vi "displayApplicationControls.vi"(10 "viewThisComponent":refnum<class "ViewThisComponent.lvclass">) -> ()   [LabVIEW 2016, in "EXAViewElements.lvlib"]
doc: "Displays application controls."
uses:
  EXAViewElements.lvlib
  ViewThisComponent/ViewThisComponent.lvclass
  home/andres/ct_cmpuserevents/ComponentTemplateCore/ComponentModel/ComponentModel/View/View.lvclass
  ComponentTemplateCore/ComponentModel/ComponentModel/Typedefs/ComponentStateValues.ctl
  Typedefs/SubDataSV.ctl
  Typedefs/EXATypedefs.lvlib
  ComponentTemplateCore/ComponentModel/ComponentModel/View/View.lvclass
panel:
  in  "Label":string(combo)
  in  "StartIsTrue":bool caption="Start"
  in  "ExitIsTrue":bool caption="Exit"
  in  "enableIsTrue":bool caption="Enable Motion"
  in  "ClearErrorIsTrue":bool caption="Clear Error"
  in  "disableIsTrue":bool caption="Disable Motion"
  in  "GoToStandbyIsTrue":bool caption="Go To Standby"
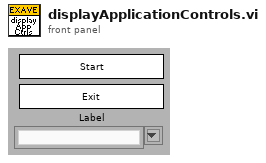
[diagram p1: front panel]
types:
  T1 = typedef "EXATypedefs.lvlib/PubDataEvents.ctl" = cluster{"DetailedState":refnum<user-event>, "ErrorCode":refnum<user-event>, "Heartbeat":refnum<user-event>, "LoopTime_ms":refnum<user-event>, "LoopTimeOutOfRange":refnum<user-event>, "RejectedCommand":refnum<user-event>, "SummaryState":refnum<user-event>, "Timestamp":refnum<user-event>, "AppliedSettingsMatchStart":refnum<user-event>, "SettingsApplied":refnum<user-event>, "SettingVersions":refnum<user-event>}
  T2 = typedef "ComponentStateValues.ctl" = enum16{"Off", "Standby", "Disabled", "Enabled", "Fault"}
  T3 = typedef "EXATypedefs.lvlib/SubDataSV.ctl" = enum16{"ClearError", "Disable", "Enable", "Exit", "GoToStandby", "HeartbeatIn", "Start"}
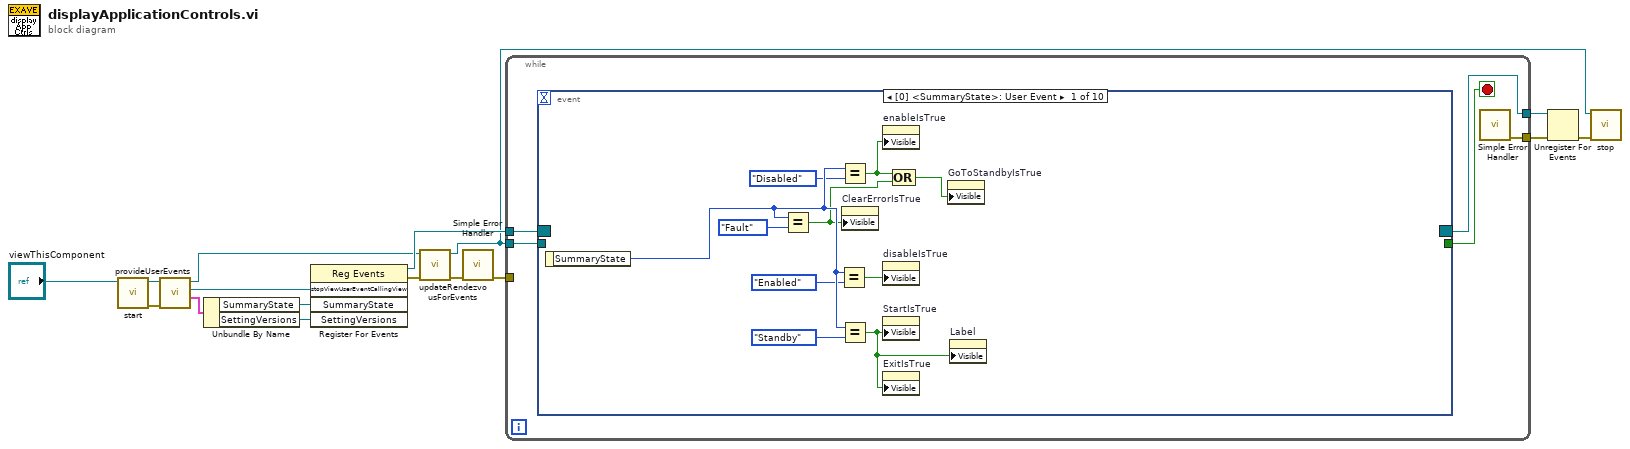
[diagram p0: block diagram]
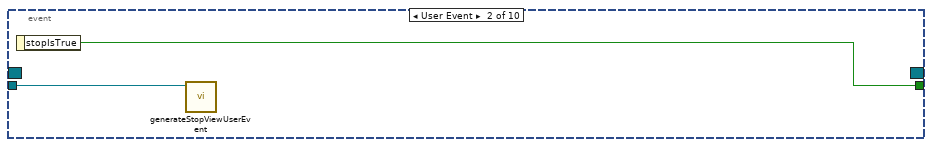
[diagram p2: hidden frame]
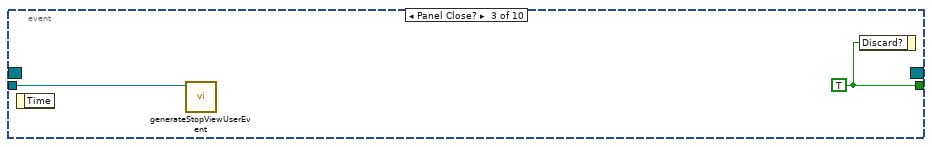
[diagram p3: hidden frame]
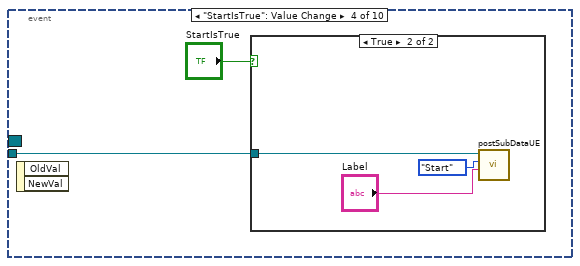
[diagram p4: hidden frame]
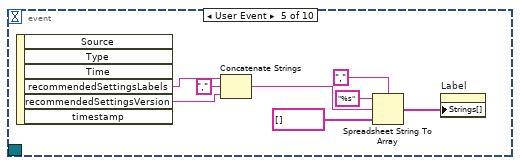
[diagram p6: hidden frame]
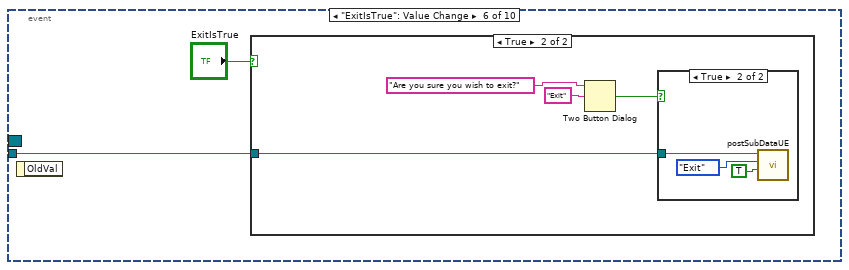
[diagram p7: hidden frame]
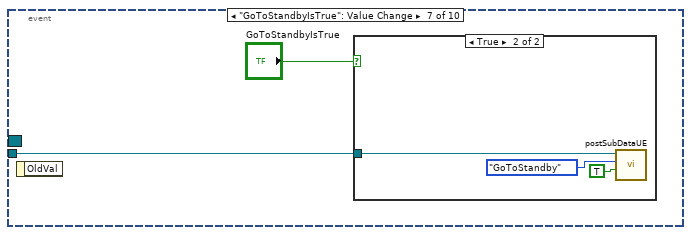
[diagram p10: hidden frame]
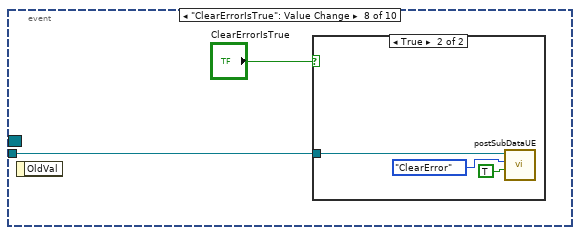
[diagram p12: hidden frame]
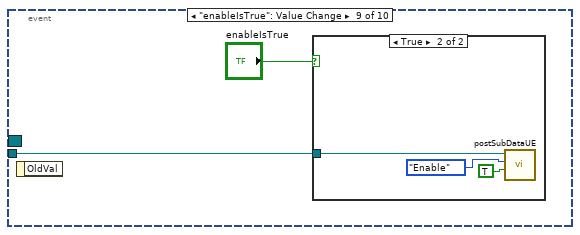
[diagram p14: hidden frame]
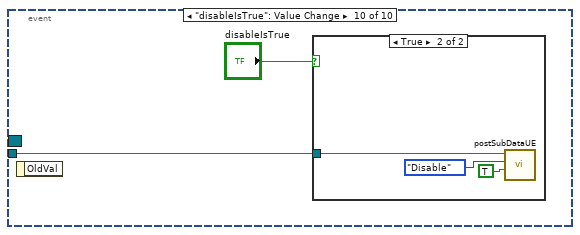
[diagram p16: hidden frame]
diagram:
  n1 = call-dynamic "start.vi"("View in"="viewThisComponent") -> ("error out"=w9:errorcluster, "View out"=w14:refnum<class "ViewThisComponent.lvclass">)  [unwired: 9 in]
  n2 = call "provideUserEvents.vi"("error in (no error)"=w9, "ViewThisComponent in"=w14) -> ("pubDataEvents"=w15:T1, "stopViewUserEventCallingView"=w16:refnum<user-event>, "ViewThisComponent out"=w3:refnum<class "ViewThisComponent.lvclass">)  [unwired: 6 in, 1 out]
  n3 = Unbundle By Name(w15) -> ("SummaryState"=w8:refnum<user-event>, "SettingVersions"=w1:refnum<user-event>)
  n4 = register-events(w16, w8, w1) -> (reference out=w12:refnum<event-registration>, error out=w5:errorcluster)  [unwired: 2 in]
  n5 = call "updateRendezvousForEvents.vi"("error in (no error)"=w5, "View in"=w3) -> ("error out"=w4:errorcluster, "View out"=w2:refnum<class "ViewThisComponent.lvclass">)  [unwired: 8 in]
  n6 = call <vilib>:"Simple Error Handler.vi"("error in (no error)"=w4) -> ("error out"=w7:errorcluster)  [unwired: 4 in, 4 out]
  n7 = while {
    tunnel: w12 -> [w21]
    tunnel: w2 -> [w20]
    tunnel: [w18] -> w10
    tunnel: w7 -> [_]
    tunnel: [w17] -> w6
    stop <- w19 stop-if-true
    n8 = event shown="[0] <SummaryState>: User Event" {
      selector: w21 -> [_ _ _ _ _ _ _ _ _ _]
      dyn-events: [_ _ _ _ _ _ _ _ _ _] -> w18
      timeout: _ -> [_ _ _ _ _ _ _ _ _ _]
      tunnel: w20 -> [_ w32 w35 w36 _ w49 w58 w63 w68 w73]
      tunnel: [_ w33 w34 _ _ _ _ _ _ _] -> w19
      event User Event {
        n9 = event-data() -> ("SummaryState"=w31:T2)  [unwired: 1 in]
        n10 = Equal?(x=w31, y=ComponentStateValues."Fault" ("componentStateValues")) -> (x = y?=w24:bool)
        n11 = Equal?(x=w31, y=ComponentStateValues."Enabled" ("componentStateValues")) -> (x = y?=w23:bool)
        n12 = Equal?(x=w31, y=ComponentStateValues."Disabled" ("componentStateValues")) -> (x = y?=w26:bool)
        n13 = Equal?(x=w31, y=ComponentStateValues."Standby" ("componentStateValues")) -> (x = y?=w22:bool)
        n14 = property on="ClearErrorIsTrue" class="Bool"("Visible"=w24) -> ()  [unwired: 2 in, 2 out]
        n15 = property on="enableIsTrue" class="Bool"("Visible"=w26) -> ()  [unwired: 2 in, 2 out]
        n16 = property on="disableIsTrue" class="Bool"("Visible"=w23) -> ()  [unwired: 2 in, 2 out]
        n17 = property on="StartIsTrue" class="Bool"("Visible"=w22) -> ()  [unwired: 2 in, 2 out]
        n18 = property on="ExitIsTrue" class="Bool"("Visible"=w22) -> ()  [unwired: 2 in, 2 out]
        n19 = Compound Arithmetic op=OR(w26, w24) -> (w25:bool)
        n20 = property on="GoToStandbyIsTrue" class="Bool"("Visible"=w25) -> ()  [unwired: 2 in, 2 out]
        n21 = property on="Label" class="CmbBox"("Visible"=w22) -> ()  [unwired: 2 in, 2 out]
      }
      event User Event {
        n22 = event-data() -> ("stopIsTrue"=w33:bool)  [unwired: 1 in]
        n23 = call "generateStopViewUserEvent.vi"("View in"=w32) -> ()  [unwired: 9 in, 2 out]
      }
      event Panel Close? {
        w34 = TRUE ("Discard?")
        n24 = event-data() -> ()  [unwired: 1 in, 1 out]
        n25 = call "generateStopViewUserEvent.vi"("View in"=w35) -> ()  [unwired: 9 in, 2 out]
        n26 = event-data("Discard?"=w34) -> ()  [unwired: 1 in, 1 out]
      }
      event "StartIsTrue": Value Change {
        n27 = event-data() -> ()  [unwired: 1 in, 2 out]
        n28 = case shown="True" "StartIsTrue" {
          tunnel: w36 -> [_ w39]
          frame False {
          }
          frame True {
            n29 = call "postSubDataUE.vi"("value"="Label", "subDataSV"=SubDataSV."Start" ("SubDataSV"), "ViewThisComponent in"=w39) -> ()  [unwired: 7 in, 2 out]
          }
        }
      }
      event User Event {
        n30 = event-data() -> ("recommendedSettingsLabels"=w44:string, "recommendedSettingsVersion"=w43:string)  [unwired: 1 in, 4 out]
        n31 = Concatenate Strings(w44, "," ("string"), w43) -> (w42:string)
        n32 = Spreadsheet String To Array(delimiter (Tab)=",", format string="%s", spreadsheet string=w42, array type (2D Dbl)=string[] []) -> (array=w45:string[])
        n33 = property on="Label" class="CmbBox"("Strings[]"=w45) -> ()  [unwired: 2 in, 2 out]
      }
      event "ExitIsTrue": Value Change {
        n34 = event-data() -> ()  [unwired: 1 in, 1 out]
        n35 = case shown="True" "ExitIsTrue" {
          tunnel: w49 -> [_ w51]
          frame False {
          }
          frame True {
            n36 = Two Button Dialog(message="Are you sure you wish to exit?", 2:"Exit" ("T button name (\"OK\")")) -> (T button?=w52:bool)  [unwired: 1 in]
            n37 = case shown="True" w52 {
              tunnel: w51 -> [_ w55]
              frame False {
              }
              frame True {
                n38 = call "postSubDataUE.vi"("value"=TRUE, "subDataSV"=SubDataSV."Exit" ("SubDataSV"), "ViewThisComponent in"=w55) -> ()  [unwired: 7 in, 2 out]
              }
            }
          }
        }
      }
      event "GoToStandbyIsTrue": Value Change {
        n39 = event-data() -> ()  [unwired: 1 in, 1 out]
        n40 = case shown="True" "GoToStandbyIsTrue" {
          tunnel: w58 -> [_ w60]
          frame False {
          }
          frame True {
            n41 = call "postSubDataUE.vi"("value"=TRUE, "subDataSV"=SubDataSV."GoToStandby" ("SubDataSV"), "ViewThisComponent in"=w60) -> ()  [unwired: 7 in, 2 out]
          }
        }
      }
      event "ClearErrorIsTrue": Value Change {
        n42 = event-data() -> ()  [unwired: 1 in, 1 out]
        n43 = case shown="True" "ClearErrorIsTrue" {
          tunnel: w63 -> [_ w65]
          frame False {
          }
          frame True {
            n44 = call "postSubDataUE.vi"("value"=TRUE ("ClearError"), "subDataSV"=SubDataSV."ClearError" ("SubDataSV"), "ViewThisComponent in"=w65) -> ()  [unwired: 7 in, 2 out]
          }
        }
      }
      event "enableIsTrue": Value Change {
        n45 = event-data() -> ()  [unwired: 1 in, 1 out]
        n46 = case shown="True" "enableIsTrue" {
          tunnel: w68 -> [_ w70]
          frame False {
          }
          frame True {
            n47 = call "postSubDataUE.vi"("value"=TRUE ("EnableMotion"), "subDataSV"=SubDataSV."Enable" ("SubDataSV"), "ViewThisComponent in"=w70) -> ()  [unwired: 7 in, 2 out]
          }
        }
      }
      event "disableIsTrue": Value Change {
        n48 = event-data() -> ()  [unwired: 1 in, 1 out]
        n49 = case shown="True" "disableIsTrue" {
          tunnel: w73 -> [_ w75]
          frame False {
          }
          frame True {
            n50 = call "postSubDataUE.vi"("value"=TRUE ("DisableMotion"), "subDataSV"=SubDataSV."Disable" ("SubDataSV"), "ViewThisComponent in"=w75) -> ()  [unwired: 7 in, 2 out]
          }
        }
      }
    }
    n51 = call <vilib>:"Simple Error Handler.vi"() -> ("error out"=w17:errorcluster)  [unwired: 5 in, 4 out]
  }
  n52 = Unregister For Events(event registration refnum=w10, error in=w6) -> (error out=w11:errorcluster)
  n53 = call-dynamic "stop.vi"("error in (no error)"=w11, "View in"=w2) -> ()  [unwired: 8 in, 2 out]
